vi "Global Tabs.vi"() -> ()   [LabVIEW 2018]
panel:
  in  "Abs-rot":bool caption="Relative"
  in  "Off-foc":dbl min=0.0 max=360.0 format="%.2f"
  in  "Off-rot":dbl min=0.0 max=360.0 format="%.2f"
  in  "Abs-foc":bool caption="Relative"
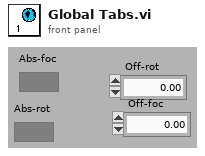
[diagram p1: front panel]
diagram:
